vi "GetStatus.vi"(8 "error in (no error)":errorcluster, 11 "AODAcq in":refnum<class "AODAcq.lvclass">) -> (0 "error out":errorcluster, 2 "Status":T2, 3 "AODAcq out":refnum<class "AODAcq.lvclass">)   [LabVIEW 2011, in "AODAcq.lvclass"]
uses:
  AODAcq.lvclass
  FPGA_Control/FPGAState.ctl
  <vilib>/Utility/error.llb/Error Cluster From Error Code.vi
  Program Files/National Instruments/LabVIEW 2011/Targets/NI/FPGA/StockFPGA_IntfPrivate/ScriptTemplates/StockFPGA_PlugInRead32.vi
  <vilib>/rvi/errors/niLvFpgaAdjustHostInterfaceError.vi
  <vilib>/rvi/interface/nirviReadWriteControl/nirviReadWriteControl.xnode
  FPGA_Control/AODRef.ctl
  FPGA_Control/FPGA Bitfiles/AODControl_FPGATarget_5751Acquire_F1CF9257.lvbitx
  FPGA_Control/AOD Control (FPGA).vi
  NiFpgaLv.dll
  <vilib>/FPGAPlugInAG/PXIe-7965R/niLvFpga_Read32_PXIe-7965R.vi
  <vilib>/rvi/interface/nirviReadWriteControl/niFpgaRWControlAccessTimeoutTemplate.vi
panel:
  out "Status.All Samples":bool
  out "Status.Update IO Missing":bool
  out "Status.TemporalChFull":bool
  out "Scan.NumPoints":u32
  out "Status.DownsampleDone":bool
  out "Status.MotionChFull":bool
  out "Status.ImChFull":bool
  out "Scan.NumMotionPoints":u32
  out "Scan.Motion Increment":u32
  out "Scan.TotalSamples":u32
  out "Debug.PMT_Unpacked_backlog":u32
  out "Debug.PMT_Data_backlog":u32
  out "AOD.UpdatesPerPoint":u32=2000
  out "Comm.CommLines":enum16{"1", "2", "4"}(ring)
  out "Comm.WriteCount":i32
  out "Comm.Written":cluster{"Address":u8, "Value":u32}[](array[cluster])
  out "Debug.Point":cluster{"X":i32, "Y":i32, "Z":i32}
  out "Status.BufferedPoints":i32
  out "Debug.PMT_Samples":u32
  out "Scan.Samples":u32
  out "Debug.PMT Array":i32[](array[numeric])
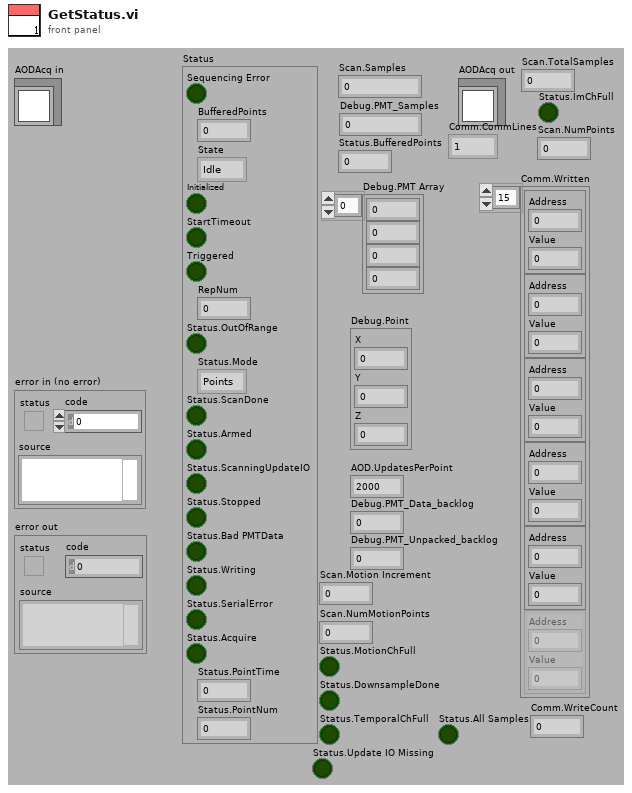
[diagram p1: front panel]
types:
  T1 = typedef "FPGAState.ctl" = enum16{"Idle", "Arm Scan", "Scan", "End Scan"}
  T2 = cluster{"Sequencing Error":bool, "BufferedPoints":i32, "State":T1, "Initialized":bool, "StartTimeout":bool, "Triggered":bool, "RepNum":u32, "Status.OutOfRange":bool, "Status.Mode":enum16{"Points", "Volume", "Idle"}, "Status.ScanDone":bool, "Status.Armed":bool, "Status.ScanningUpdateIO":bool, "Status.Stopped":bool, "Status.Bad PMTData":bool, "Status.Writing":bool, "Status.SerialError":bool, "Status.Acquire":bool, "Status.PointTime":u32, "Status.PointNum":u64}
  T3 = typedef "AODRef.ctl" = refnum<k20>
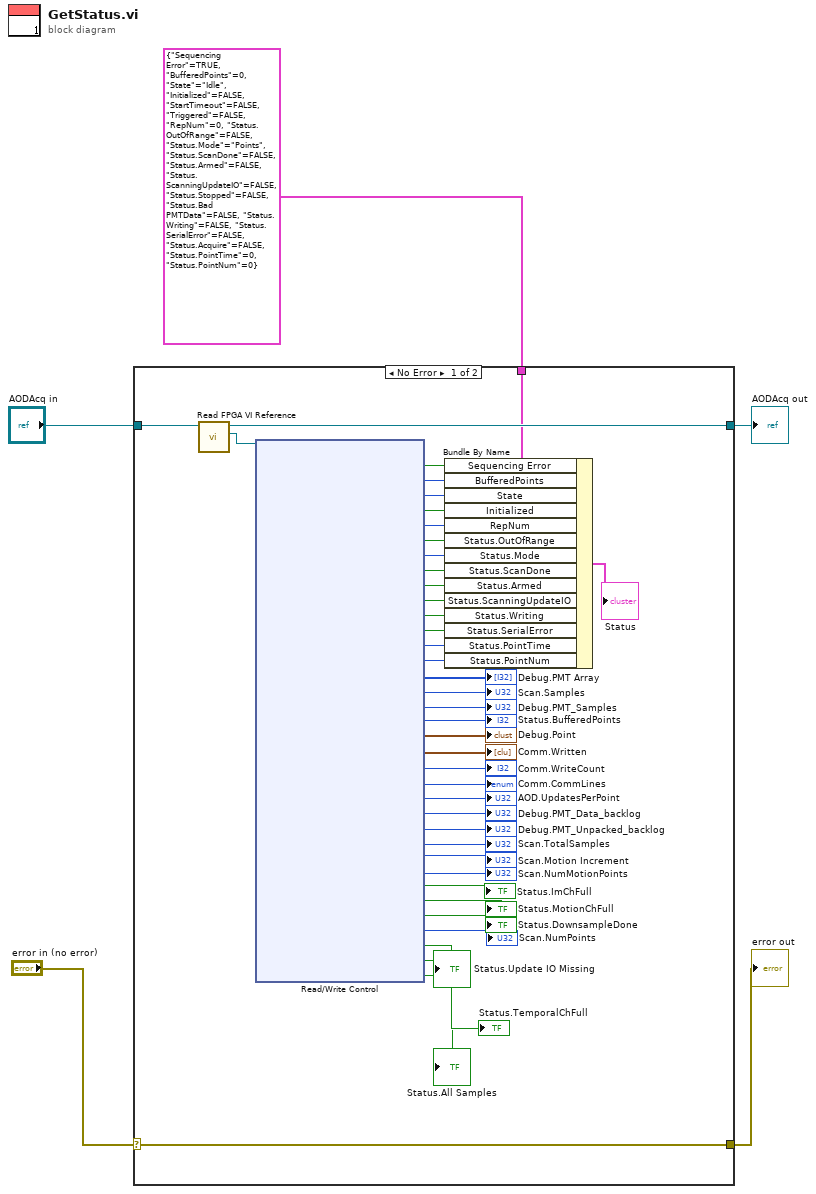
[diagram p0: block diagram]
diagram:
  n1 = case shown="No Error" "error in (no error)" {
    selector: "error in (no error)" -> [w46 w48]
    tunnel: [w46 w48] -> w4
    tunnel: [w44 w47] -> w2
    tunnel: "AODAcq in" -> [w45 w47]
    tunnel: T2 {"Sequencing Error"=TRUE, "BufferedPoints"=0, "State"=enum."Idle", "Initialized"=FALSE, "StartTimeout"=FALSE, "Triggered"=FALSE, "RepNum"=0, "Status.OutOfRange"=FALSE, "Status.Mode"=enum."Points", "Status.ScanDone"=FALSE, "Status.Armed"=FALSE, "Status.ScanningUpdateIO"=FALSE, "Status.Stopped"=FALSE, "Status.Bad PMTData"=FALSE, "Status.Writing"=FALSE, "Status.SerialError"=FALSE, "Status.Acquire"=FALSE, "Status.PointTime"=0, "Status.PointNum"=0} -> [w40 _]
    frame No Error {
      n2 = call-dynamic "Read FPGA VI Reference.vi"("AODAcq in"=w45) -> ("FPGA VI Reference"=w43:T3, "AODAcq out"=w44:refnum<class "AODAcq.lvclass">)  [unwired: 8 in, 1 out]
      n3 = xnode "Read/Write Control"("FPGA VI Reference In"=w43) -> ("Status.Sequencing error"=w42:bool, "Status.BufferedPoints"=w41:i32, "Status.State"=w39:T1, "Status.Initialized"=w38:bool, "Status.RepNum"=w37:u32, "Status.OutOfRange"=w36:bool, "Status.Mode"=w35:enum16{"Points", "Volume", "Idle"}, "Status.ScanDone"=w34:bool, "Status.Armed"=w33:bool, "Status.ScanUpdateIO"=w32:bool, "Status.Writing"=w29:bool, "Status.Serial error"=w8:bool, "Status.PointTime"=w30:u32, "Status.PointNum"=w31:u32, "Debug.PMT Array"=→"Debug.PMT Array":i32[], "Scan.Samples"=→"Scan.Samples":u32, "Debug.PMT_Samples"=→"Debug.PMT_Samples":u32, "Status.BufferedPoints"=→"Status.BufferedPoints":i32, "Debug.Point"=→"Debug.Point":cluster{"X":i32, "Y":i32, "Z":i32}, "Comm.Written"=→"Comm.Written":cluster{"Address":u8, "Value":u32}[], "Comm.WritenCount"=→"Comm.WriteCount":i32, "Comm.CommLines"=→"Comm.CommLines":enum16{"1", "2", "4"}, "AOD.UpdatesPerPoint"=→"AOD.UpdatesPerPoint":u32, "Debug.PMT_Data_backlog"=→"Debug.PMT_Data_backlog":u32, "Debug.PMT_Unpacked_backlog"=→"Debug.PMT_Unpacked_backlog":u32, "Scan.TotalSamples"=→"Scan.TotalSamples":u32, "Scan.Motion Increment"=→"Scan.Motion Increment":u32, "Scan.NumMotionPoints"=→"Scan.NumMotionPoints":u32, "Status.ImChFull"=→"Status.ImChFull":bool, "Status.MotionChFull"=→"Status.MotionChFull":bool, "Status.DownsampleDone"=→"Status.DownsampleDone":bool, "Scan.NumPoints"=→"Scan.NumPoints":u32, "Status.TemporalChFull"=→"Status.TemporalChFull":bool, "Status.Update IO Missing"=→"Status.Update IO Missing":bool, "Status.All Samples"=→"Status.All Samples":bool)  [unwired: 1 in, 2 out]
      n4 = Bundle By Name(cluster=w40, "Sequencing Error"=w42, "BufferedPoints"=w41, "State"=w39, "Initialized"=w38, "RepNum"=w37, "Status.OutOfRange"=w36, "Status.Mode"=w35, "Status.ScanDone"=w34, "Status.Armed"=w33, "Status.ScanningUpdateIO"=w32, "Status.Writing"=w29, "Status.SerialError"=w8, "Status.PointTime"=w30, "Status.PointNum"=w31) -> (→"Status":T2)
    }
    frame Error {
    }
  }
  "error out" <- w4
  "AODAcq out" <- w2
